vi "Release.vi"(10 "Self Queue":refnum<data-value>) -> (0 "error out":errorcluster, 2 "Remaining":refnum<class "Msg Strategy.lvclass">[](array[class]))   [LabVIEW 2021, in "jettl.lvlib" / "Self Queue.lvlib"]
uses:
  Self Queue.lvlib
  Msg Strategy/Msg Strategy.lvclass
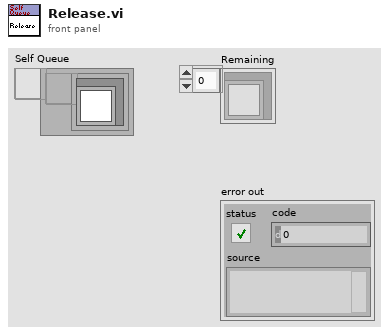
[diagram p1: front panel]
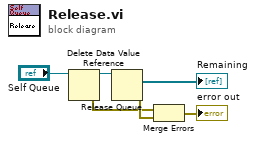
[diagram p0: block diagram]
diagram:
  n1 = Delete Data Value Reference(data value reference="Self Queue") -> (data value=w6:refnum<queue>, error out=w3:errorcluster)  [unwired: 1 in]
  n2 = Release Queue(queue=w6) -> (remaining elements=→"Remaining":refnum<class "Msg Strategy.lvclass">[], error out=w5:errorcluster)  [unwired: 2 in, 1 out]
  n3 = Merge Errors(w3, w5) -> (→"error out":errorcluster)
